vi "RSZVB Set Two Port Transmission Coefficients Enabled.vi"(8 "error in (no error)":errorcluster {"code" format="%.0x"}, 9 "Two-Port Enabled (Off)":bool, 11 "VISA session":refnum<visa-resource-name>) -> (0 "error out":errorcluster {"code" format="%.0x"}, 3 "dup VISA session":refnum<visa-resource-name>)   [LabVIEW 2011]
doc: "This VI enables or disables the use of two-port transmission coefficients. \n\nNotes:\n(1) The power loss list must contain at least one point before the transmission coefficients can be enabled.\n\nRemote-control command(s):\nSOURce<Ch>:POWer<Pt>:CORRection:TCOefficient[:STATe] <Boolean>"
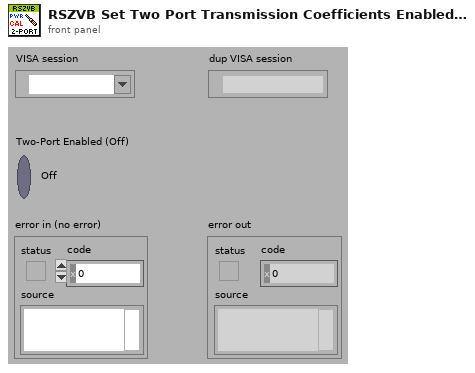
[diagram p1: front panel]
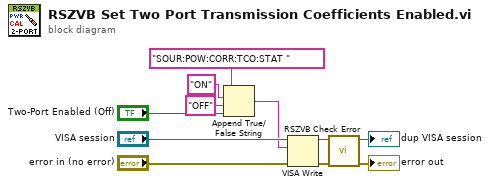
[diagram p0: block diagram]
diagram:
  n1 = Append True/False String(1:"Two-Port Enabled (Off)", 2:"OFF" ("false string"), 3:"ON" ("true string"), 4:"SOUR:POW:CORR:TCO:STAT " ("string (\"\")")) -> (0:w1:string)
  n2 = VISA Write(VISA resource name="VISA session", write buffer=w1, error in (no error)="error in (no error)") -> (VISA resource name out=w7:refnum<visa-resource-name>, error out=w8:errorcluster)  [unwired: 1 out]
  n3 = call "RSZVB Check Error.vi"("error in (no error)"=w8, "VISA session"=w7) -> ("error out"=→"error out":errorcluster, "dup VISA session"=→"dup VISA session":refnum<visa-resource-name>)  [unwired: 8 in]
